vi "Configure.vi"(8 "error in (no error)":errorcluster, 11 "DAQCascade512 in":refnum<class "DAQCascade512.lvclass">) -> (0 "error out":errorcluster, 2 "cancelled?":bool, 3 "DAQCascade512 out":refnum<class "DAQCascade512.lvclass">)   [LabVIEW 2012, in "DAQCascade512.lvclass"]
doc: "The configure method configures the details for the RabbitMQ connection, the observers and the mapping script.\n\nIn the derived class, make a call to the parent for setting these parameters."
uses:
  DAQCascade512.lvclass
  OLD_apparatus_VI/VI/Image_type.ctl
  DAQCascade512.lvclass/DAQCascade512.ctl
  <vilib>/Distrio/Murmex/Murmex/Murmex.lvclass
panel:
  in  "Image type":T1=6 items=["8 bit signed"=1, "16 bit signed"=2, "32 bit signed"=3, "32 bit floating"=4, "64 bit floating"=5, "8 bit unsigned"=6, "16 bit unsigned"=7, "32 bit unsigned"=8]
  in  "temperature":dbl
  in  "button:\"call parent\"":bool
  in  "button:\"ok\"":bool
  in  "button:cancel":bool
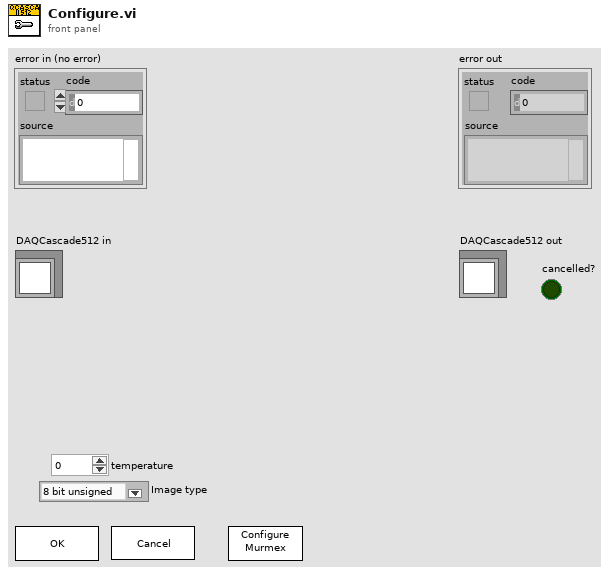
[diagram p1: front panel]
types:
  T1 = typedef "Image_type.ctl" = u32
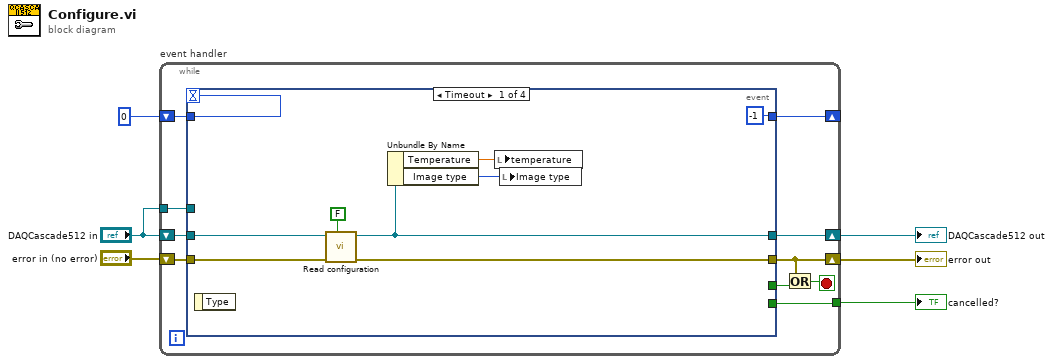
[diagram p0: block diagram]
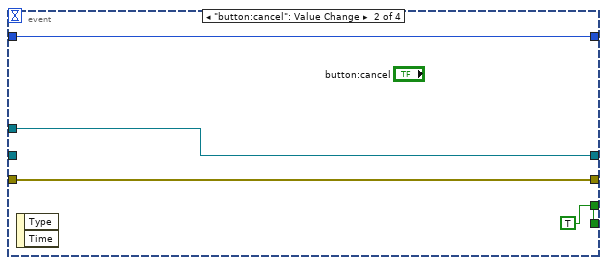
[diagram p2: hidden frame]
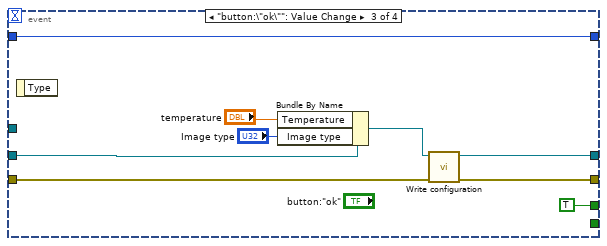
[diagram p3: hidden frame]
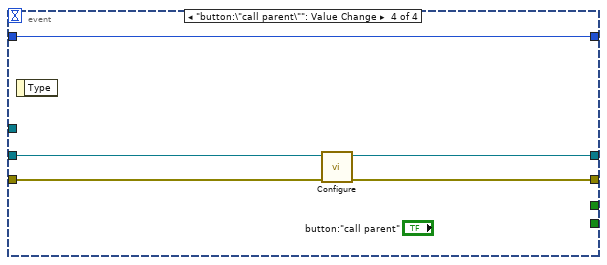
[diagram p4: hidden frame]
diagram:
  n1 = while "event handler" {
    shift-right: [w16] -> _
    shift-left: 0 -> [w12]
    shift-right: [w15] -> w4
    shift-left: "DAQCascade512 in" -> [w11]
    tunnel: [w10] -> w3
    shift-right: [w14] -> w5
    shift-left: "error in (no error)" -> [w8]
    tunnel: "DAQCascade512 in" -> [w7]
    stop <- w13 stop-if-true
    n2 = event shown="[0] Timeout" {
      selector: _ -> [_ _ _ _]
      dyn-events: _ -> [_ _ _ _]
      timeout: w12 -> [_ _ _ _]
      tunnel: w12 -> [_ w28 w30 w38]
      tunnel: [-1 w28 w30 w38] -> w16
      tunnel: w11 -> [w23 _ w34 w42]
      tunnel: [w22 w26 w37 w40] -> w14
      tunnel: [w20 w25 w35 w39] -> w15
      tunnel: w7 -> [_ w25 _ _]
      tunnel: [_ w27 TRUE _] -> w9
      tunnel: [_ w27 _ _] -> w10
      tunnel: w8 -> [w19 w26 w36 w41]
      event Timeout {
        n3 = event-data() -> ()  [unwired: 1 in, 1 out]
        n4 = call-dynamic "Read configuration.vi"("force loading?"=FALSE, "error in (no error)"=w19, "DAQCascade512 in"=w23) -> ("error out"=w22:errorcluster, "DAQCascade512 out"=w20:refnum<class "DAQCascade512.lvclass">)  [unwired: 7 in]
        n5 = Unbundle By Name(w20) -> ("Temperature"=w18:dbl, "Image type"=w17:T1)
        n6 = local write "temperature"(w18) -> ()
        n7 = local write "Image type"(w17) -> ()
      }
      event "button:cancel": Value Change {
        w27 = TRUE
        n8 = event-data() -> ()  [unwired: 1 in, 2 out]
      }
      event "button:\"ok\"": Value Change {
        n9 = event-data() -> ()  [unwired: 1 in, 1 out]
        n10 = Bundle By Name(cluster=w34, "Temperature"="temperature", "Image type"="Image type") -> (w33:refnum<class "DAQCascade512.lvclass">)
        n11 = call-dynamic "Write configuration.vi"("error in (no error)"=w36, "DAQCascade512 in"=w33) -> ("error out"=w37:errorcluster, "DAQCascade512 out"=w35:refnum<class "DAQCascade512.lvclass">)  [unwired: 8 in]
      }
      event "button:\"call parent\"": Value Change {
        n12 = event-data() -> ()  [unwired: 1 in, 1 out]
        n13 = call-parent "Configure.vi"("error in (no error)"=w41, "Murmex in"=w42) -> ("error out"=w40:errorcluster, "Murmex out"=w39:refnum<class "DAQCascade512.lvclass">)  [unwired: 7 in, 1 out]
      }
    }
    n14 = Or(x=w14, y=w9) -> (x .or. y?=w13:bool)
  }
  "error out" <- w5
  "DAQCascade512 out" <- w4
  "cancelled?" <- w3
